vi "ReadMoxa12.vi"(0 "PORT 1":dbl, 1 "PORT 6":dbl, 2 "PORT 7":dbl, 3 "PORT 8":dbl, 4 "PORT12":dbl, 5 "PORT 2":dbl, 7 "PORT 3":dbl, 9 "PORT 4":dbl, 11 "PORT 5":dbl, 12 "PORT 9":dbl, 13 "PORT 10":dbl, 14 "PORT 11":dbl) -> (6 "params":dbl[](array[numeric]))   [LabVIEW 2017]
uses:
  BERTTA.dll
panel:
  # "int ports[12] = {1,2,4,3,6,5,8,0,0,0,0,0};"
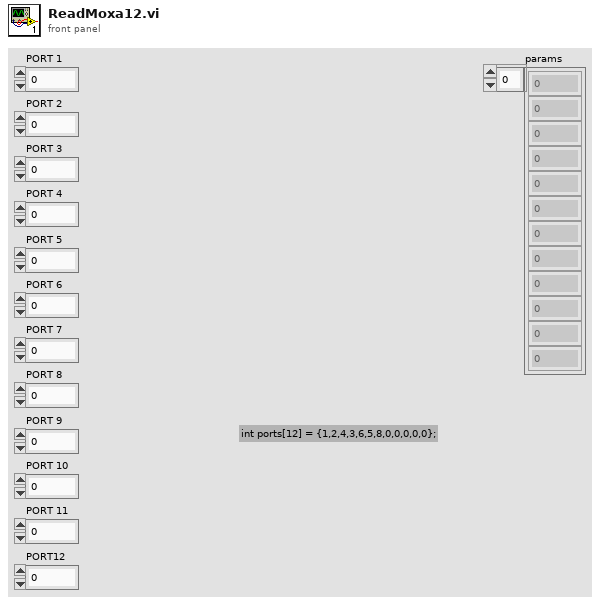
[diagram p1: front panel]
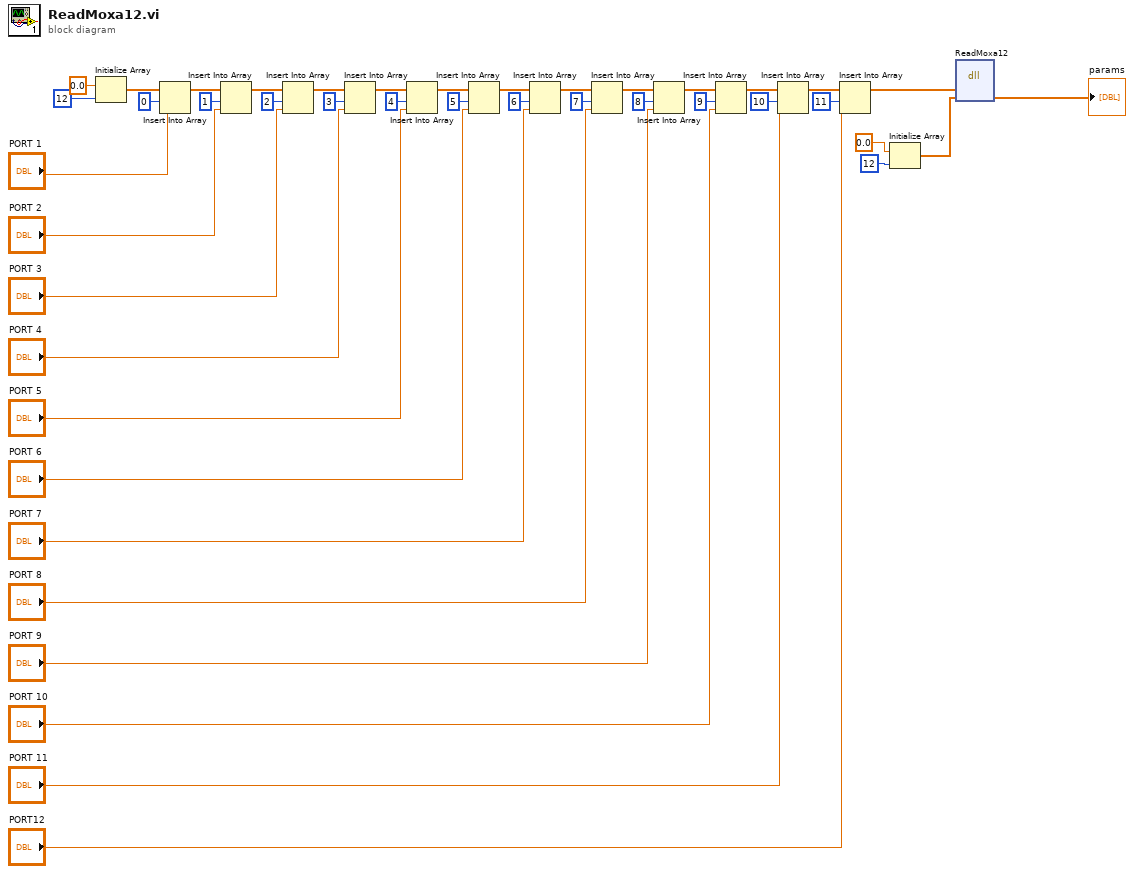
[diagram p0: block diagram]
diagram:
  n1 = Initialize Array(0.0 ("element"), 12 ("dimension size")) -> (w42:dbl[])
  n2 = Insert Into Array(array=w42, index=0, new element="PORT 1") -> (w40:dbl[])
  n3 = Insert Into Array(array=w40, index=1, new element="PORT 2") -> (w39:dbl[])
  n4 = Insert Into Array(array=w39, index=2, new element="PORT 3") -> (w38:dbl[])
  n5 = Insert Into Array(array=w38, index=3, new element="PORT 4") -> (w37:dbl[])
  n6 = Insert Into Array(array=w37, index=4, new element="PORT 5") -> (w36:dbl[])
  n7 = Insert Into Array(array=w36, index=5, new element="PORT 6") -> (w35:dbl[])
  n8 = Insert Into Array(array=w35, index=6, new element="PORT 7") -> (w34:dbl[])
  n9 = Insert Into Array(array=w34, index=7, new element="PORT 8") -> (w33:dbl[])
  n10 = Insert Into Array(array=w33, index=8, new element="PORT 9") -> (w32:dbl[])
  n11 = Insert Into Array(array=w32, index=9, new element="PORT 10") -> (w31:dbl[])
  n12 = Insert Into Array(array=w31, index=10, new element="PORT 11") -> (w30:dbl[])
  n13 = Insert Into Array(array=w30, index=11, new element="PORT12") -> (w29:dbl[])
  n14 = Initialize Array(0.0 ("element"), 12 ("dimension size")) -> (w2:dbl[])
  n15 = dll-call lib="C:/Users/shresplab/OneDrive - Kemira Oyj/Documents/GitHub/Bertta/BERTTA/x64/Debug/BERTTA.dll" fn="ReadMoxa12"("ports"=w29, "params"=w2) -> ("params"=→"params":dbl[])  [unwired: 5 in, 2 out]
